vi "dfd_Font Control.vi"(10 "tpye":u16(ring) items=["Number Font", "Variable Font", "Script Font"], 11 "fonts input":T2(array[cluster])) -> (3 "font output":T1={"Font Name:"="Application Font", "Size"=12, "Strikeout?"=FALSE, "Italic?"=FALSE, "Underline?"=FALSE, "Outline?"=TRUE, "Shadow?"=FALSE, "Bold?"=TRUE})   [LabVIEW 2017, in "NI_DigFilter_Process.lvlib"]
uses:
  <vilib>/addons/Digital Filter Design/NI_DigFilter_Process.lvlib
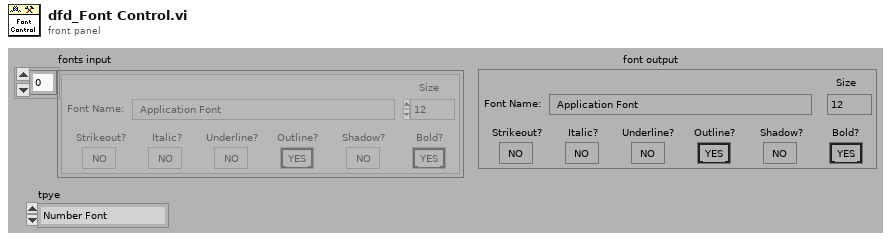
[diagram p1: front panel]
types:
  T1 = cluster{"Font Name:":string, "Size":i16, "Strikeout?":bool, "Italic?":bool, "Underline?":bool, "Outline?":bool, "Shadow?":bool, "Bold?":bool}
  T2 = cluster{"Font Name:":string, "Size":i16, "Strikeout?":bool, "Italic?":bool, "Underline?":bool, "Outline?":bool, "Shadow?":bool, "Bold?":bool}[]
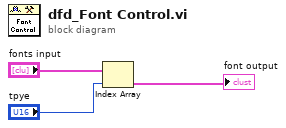
[diagram p0: block diagram]
diagram:
  n1 = Index Array(array="fonts input", index="tpye") -> (element=→"font output":T1)
